vi "Print Image.vi"(10 "Images":T1[](array[typedef]), 11 "Path":path=path "C:/Users/telsey/Desktop/Personal Projects/Photobooth/Photos") -> (3 "New Image Path":path)   [LabVIEW 2012]
uses:
  <vilib>/vision/Image Controls.llb/IMAQ Image.ctl
  Image States.ctl
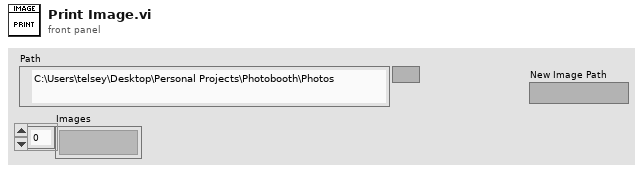
[diagram p1: front panel]
types:
  T1 = typedef "IMAQ Image.ctl" = refnum<image>
  T2 = typedef "Image States.ctl" = enum16{"Init", "Print"}
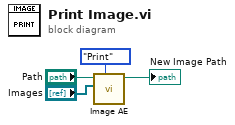
[diagram p0: block diagram]
diagram:
  n1 = call "Image AE.vi"("Image State"=Image_States."Print", "Images"="Images", "Path"="Path") -> ("New Image Path"=→"New Image Path":path)  [unwired: 8 in]
